vi "FTW-Ether-CreateEndpoint.vi"(5 "Endpoint Type":T2, 7 "Message Transport Scheme":T1, 11 "error in":errorcluster) -> (4 "FTW Endpoint":refnum<class "FTW-Endpoint.lvclass">, 15 "error out":errorcluster)   [LabVIEW 2015, in "FTW-Ether.lvclass"]
uses:
  FTW-Ether.lvclass
  Endpoint/FTW-Endpoint.lvclass
  FTW-Ether-EndpointType.ctl
  FTW-Ether-MessageTransportScheme.ctl
  TCP/FTW-Endpoint-TCP.lvclass
panel:
  # "Inputs"
  # "Outputs"
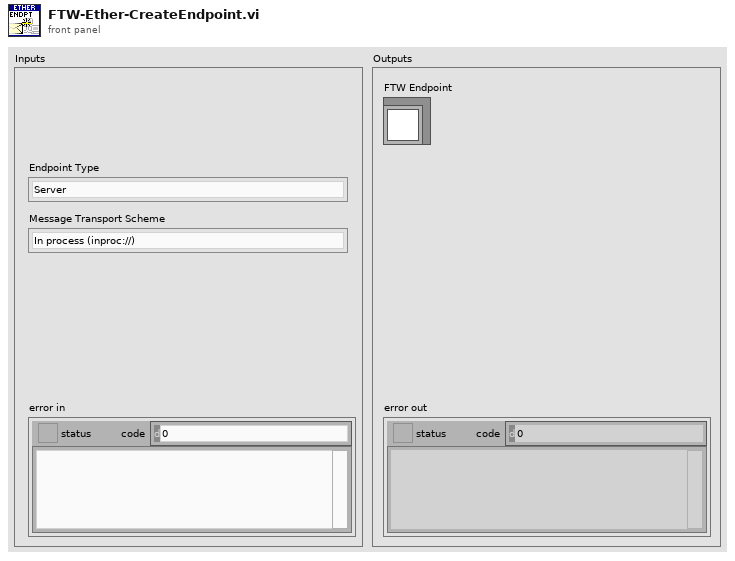
[diagram p1: front panel]
types:
  T1 = typedef "FTW-Ether.lvclass/FTW-Ether-MessageTransportScheme.ctl" = enum16{"In process (inproc://)", "TCP (tcp://)"}
  T2 = typedef "FTW-Ether.lvclass/FTW-Ether-EndpointType.ctl" = enum16{"Server", "Client", "Publisher", "Subscriber"}
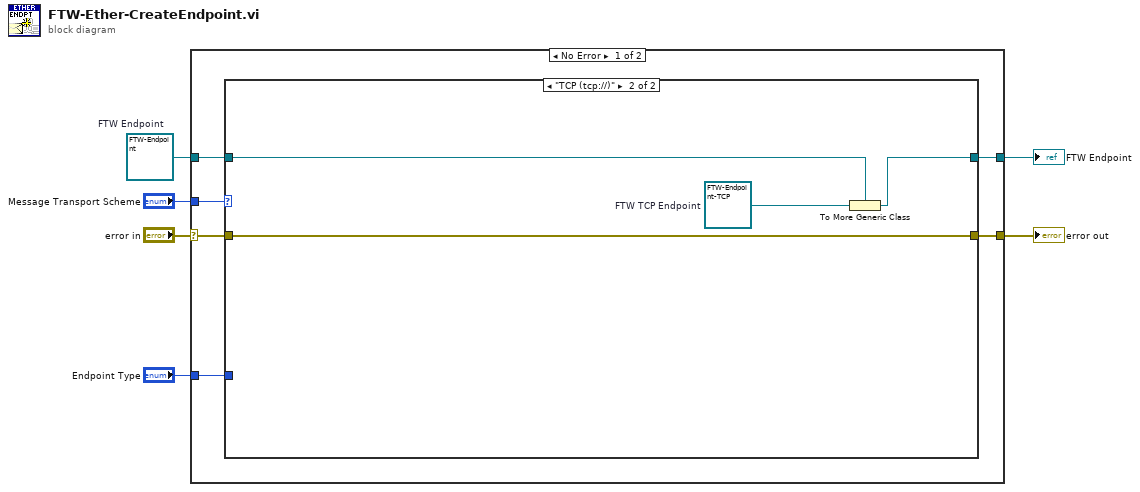
[diagram p0: block diagram]
diagram:
  w1 = refnum<class "FTW-Endpoint.lvclass"> refnum  # FTW Endpoint
  n1 = case shown="No Error" "error in" {
    selector: "error in" -> [w9 w20]
    tunnel: [w12 w19] -> w6
    tunnel: [w11 w20] -> w5
    tunnel: "Message Transport Scheme" -> [w10 _]
    tunnel: "Endpoint Type" -> [w8 _]
    tunnel: w1 -> [w7 w19]
    frame No Error {
      n2 = case shown="\"TCP (tcp://)\"" w10 {
        tunnel: [w14 w16] -> w12
        tunnel: [w13 w18] -> w11
        tunnel: w9 -> [w13 w18]
        tunnel: w8 -> [_ _]
        tunnel: w7 -> [w14 w17]
        frame "In process (inproc://)" {
        }
        frame "TCP (tcp://)" {
          w15 = refnum<class "FTW-Endpoint-TCP.lvclass"> refnum  # FTW TCP Endpoint
          n3 = To More Generic Class(target class=w17, reference=w15) -> (generic class reference=w16:refnum<class "FTW-Endpoint.lvclass">)
        }
      }
    }
    frame Error {
    }
  }
  "error out" <- w5
  "FTW Endpoint" <- w6
